vi "stage track by AO.vi"(5 "t":dbl, 7 "speed":dbl, 8 "error in":errorcluster, 9 "B":dbl, 10 "A":dbl, 11 "XPS Reference IN":refnum<k24>) -> (0 "error out":errorcluster, 2 "stage Y":refnum<k21>, 3 "XPS Reference OUT":refnum<k24>)   [LabVIEW 2015]
uses:
  D:/labview program/whole brain TP_220607/sub vi/XPS-UNIFIED/LabVIEW VIs/LabVIEW Source Code/Dll/Newport.XPS.CommandInterface.dll
  XPS-UNIFIED/LabVIEW VIs/LabVIEW Source Code/Dll/Newport.XPS.CommandInterface.dll
  <vilib>/DAQmx/write.llb/DAQmx Write (Analog 1D DBL 1Chan NSamp).vi
  <vilib>/DAQmx/create/channels.llb/DAQmx Create Channel (AO-Voltage-Basic).vi
  <vilib>/DAQmx/configure/timing.llb/DAQmx Timing (Sample Clock).vi
  <vilib>/DAQmx/configure/trigger.llb/DAQmx Start Trigger (Digital Edge).vi
  <vilib>/DAQmx/miscellaneous.llb/DAQmx Fill In Error Info.vi
panel:
  in  "rate":dbl=1000.0 format="%#_13g"
  out "Waveform Graph":dbl[](graph)
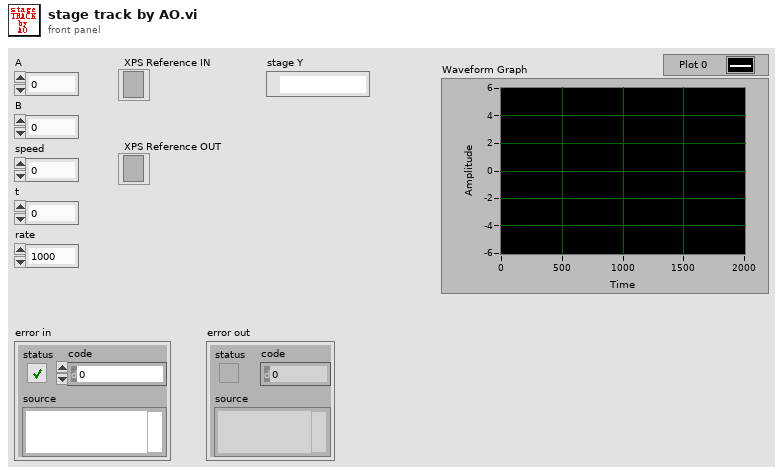
[diagram p1: front panel]
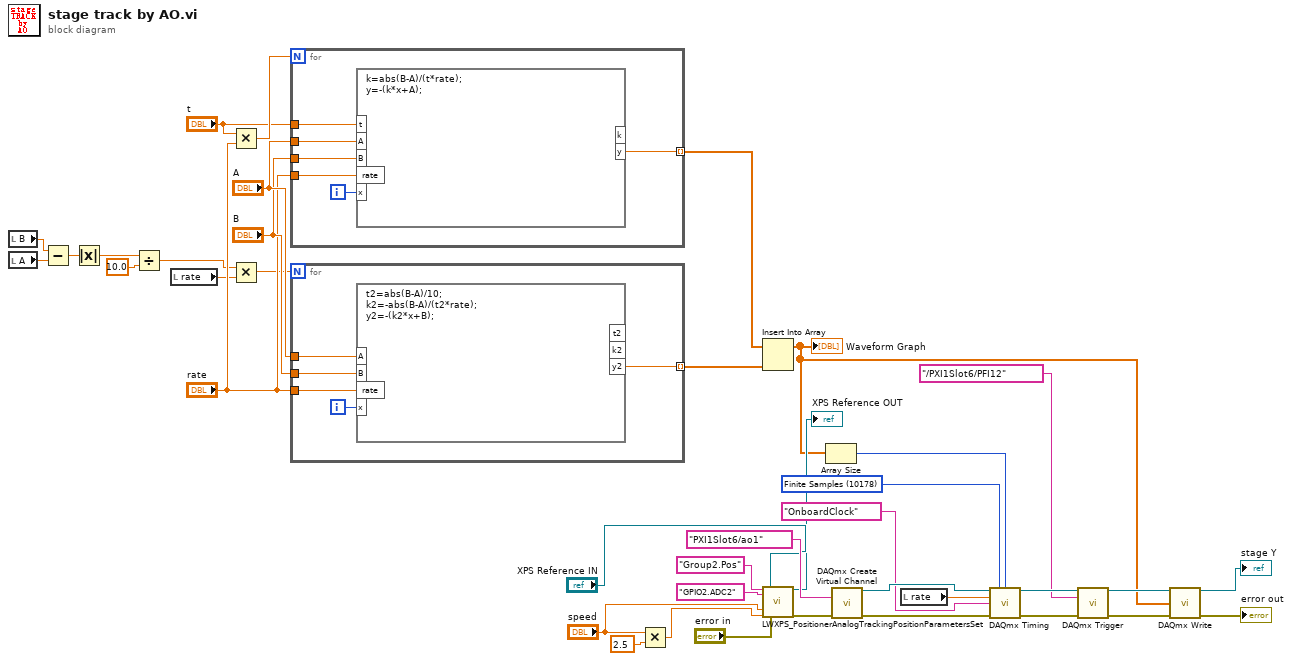
[diagram p0: block diagram]
diagram:
  w23 = 10178 items=["Finite Samples"=10178, "Continuous Samples"=10123, "Hardware Timed Single Point"=12522] ("sample mode")
  n1 = local read "B"() -> (w11:dbl)
  n2 = local read "A"() -> (w10:dbl)
  n3 = Subtract(x=w11, y=w10) -> (x-y=w9:dbl)
  n4 = Absolute Value(x=w9) -> (abs(x)=w8:dbl)
  n5 = Divide(x=w8, y=10.0) -> (x/y=w6:dbl)
  n6 = local read "rate"() -> (w5:dbl)
  n7 = Multiply(x="t", y="rate") -> (x*y=w19:dbl)
  n8 = Multiply(x=w6, y=w5) -> (x*y=w4:dbl)
  n9 = for {
    N: w19 -> [_]
    tunnel: "A" -> [w45]
    tunnel: "B" -> [w44]
    tunnel: "rate" -> [w43]
    tunnel: [w40] -> w3 mode=indexing
    tunnel: "t" -> [w41]
    i -> [w42]
    n10 = formula code="k=abs(B-A)/(t*rate);\ny=-(k*x+A);"("A"=w45, "B"=w44, "rate"=w43, "x"=w42, "t"=w41) -> ("y"=w40:dbl)  [unwired: 1 out]
  }
  n11 = for {
    N: w4 -> [_]
    tunnel: "A" -> [w50]
    tunnel: [w48] -> w2 mode=indexing
    tunnel: "B" -> [w47]
    tunnel: "rate" -> [w46]
    i -> [w49]
    n12 = formula code="t2=abs(B-A)/10;\nk2=-abs(B-A)/(t2*rate);\ny2=-(k2*x+B);"("A"=w50, "B"=w47, "rate"=w46, "x"=w49) -> ("y2"=w48:dbl)  [unwired: 2 out]
  }
  n13 = Multiply(x="speed", y=2.5) -> (x*y=w34:dbl)
  n14 = Insert Into Array(array=w3, new element=w2) -> (w1:dbl[])  [unwired: 1 in]
  "Waveform Graph" <- w1
  n15 = call "LWXPS_PositionerAnalogTrackingPositionParametersSet.vi"("Positioner Name"="Group2.Pos", "Analog input name"="GPIO2.ADC2", "Velocity"="speed", "Acceleration"=w34, "CommandInterfaceXPS.XPS"="XPS Reference IN", "LabVIEW error IN"="error in") -> ("CommandInterfaceXPS.XPS"=→"XPS Reference OUT":refnum<k24>, "LabVIEW error OUT"=w27:errorcluster)  [unwired: 10 in, 2 out]
  n16 = Array Size(array=w1) -> (size(s)=w17:i32)
  n17 = call-poly <vilib>:"DAQmx Create Virtual Channel.vi"("physical channels"=tag "PXI1Slot6/ao1" ("Physical Channel(s)"), "error in"=w27) -> ("task out"=w33:refnum<k21>, "error out"=w32:errorcluster)  [unwired: 12 in]
  n18 = local read "rate"() -> (w18:dbl)
  n19 = call-poly <vilib>:"DAQmx Timing.vi"("task/channels in"=w33, "sample mode"=w23, "samples per channel"=w17, "rate"=w18, "source"=tag "OnboardClock", "error in"=w32) -> ("task out"=w31:refnum<k21>, "error out"=w30:errorcluster)  [unwired: 8 in]
  n20 = call-poly <vilib>:"DAQmx Trigger.vi"("task/channels in"=w31, "source"=tag "/PXI1Slot6/PFI12", "error in"=w30) -> ("task out"=w29:refnum<k21>, "error out"=w28:errorcluster)  [unwired: 11 in]
  n21 = call-poly <vilib>:"DAQmx Write.vi"("task/channels in"=w29, "data"=w1, "error in"=w28) -> ("task out"=→"stage Y":refnum<k21>, "error out"=→"error out":errorcluster)  [unwired: 10 in, 1 out]
